vi "HFRR ADV v07.vi"() -> ()   [LabVIEW 2025] (continued)
, 1.5097292153342525, 1.5111107672344057, 1.5104967441676709, 1.5138738710347124, 1.5138738710347124, 1.5124923191345592, 1.5115712845344569, 1.510957261467722, 1.509422203800885, 1.5108037557010383, 1.5104967441676709, 1.5101897326343034, 1.5104967441676709, 1.5101897326343034, 1.5101897326343034, 1.5103432384009872, 1.5101897326343034, 1.5104967441676709, 1.5101897326343034, 1.5108037557010383, 1.5106502499343546, 1.5098827211009362, 1.5112642730010895, 1.5098827211009362, 1.510957261467722, 1.5104967441676709, 1.5101897326343034, 1.5101897326343034, 1.5103432384009872, 1.5108037557010383, 1.5097292153342525, 1.5111107672344057, 1.5108037557010383, 1.5104967441676709, 1.5112642730010895, 1.5103432384009872, 1.5097292153342525, 1.5104967441676709, 1.5106502499343546, 1.5108037557010383, 1.5100362268676197, 1.5106502499343546, 1.5106502499343546, 1.5103432384009872, 1.5097292153342525, 1.5106502499343546, 1.5100362268676197, 1.5111107672344057, 1.5108037557010383, 1.5100362268676197, 1.5101897326343034, 1.5117247903011406, 1.5117247903011406, 1.510957261467722, 1.5100362268676197, 1.510957261467722, 1.5112642730010895, 1.5103432384009872, 1.5112642730010895, 1.5098827211009362, 1.5112642730010895, 1.510957261467722, 1.5106502499343546, 1.5123388133678755, 1.5123388133678755, 1.5103432384009872, 1.5101897326343034, 1.5101897326343034, 1.5104967441676709, 1.5097292153342525, 1.5111107672344057, 1.5108037557010383, 1.5126458249012429, 1.5117247903011406, 1.5100362268676197, 1.5106502499343546, 1.5098827211009362, 1.5104967441676709, 1.5098827211009362, 1.5106502499343546, 1.5115712845344569, 1.5108037557010383, 1.5112642730010895, 1.5100362268676197, 1.5112642730010895, 1.5104967441676709, 1.5098827211009362, 1.5091151922675177, 1.5112642730010895, 1.5103432384009872, 1.514641399868131, 1.5154089287015495, 1.5117247903011406, 1.5111107672344057, 1.5101897326343034, 1.5098827211009362, 1.5106502499343546, 1.5106502499343546, 1.5106502499343546, 1.5106502499343546, 1.5104967441676709, 1.5112642730010895, 1.5103432384009872, 1.5108037557010383, 1.5106502499343546, 1.5097292153342525, 1.510957261467722, 1.5112642730010895, 1.5103432384009872, 1.510957261467722, 1.5112642730010895, 1.5111107672344057, 1.5106502499343546, 1.5097292153342525, 1.5101897326343034, 1.5097292153342525, 1.5114177787677732, 1.5100362268676197, 1.5103432384009872, 1.5114177787677732, 1.5104967441676709, 1.5112642730010895, 1.5108037557010383, 1.509422203800885, 1.5108037557010383, 1.510957261467722, 1.5108037557010383, 1.5108037557010383, 1.5106502499343546, 1.5108037557010383, 1.510957261467722, 1.5117247903011406, 1.5092686980342014, 1.5098827211009362, 1.5108037557010383, 1.5104967441676709, 1.510957261467722, 1.5111107672344057, 1.5114177787677732, 1.5114177787677732, 1.5114177787677732, 1.5100362268676197, 1.509422203800885, 1.5114177787677732, 1.5106502499343546, 1.5100362268676197, 1.5108037557010383, 1.5103432384009872, 1.5108037557010383, 1.510957261467722, 1.5101897326343034, 1.5103432384009872, 1.5098827211009362, 1.5114177787677732, 1.5108037557010383, 1.5104967441676709, 1.510957261467722, 1.5101897326343034, 1.5111107672344057, 1.5106502499343546, 1.5103432384009872, 1.5108037557010383, 1.5095757095675688, 1.5106502499343546, 1.5103432384009872, 1.5104967441676709, 1.5111107672344057, 1.5104967441676709, 1.5103432384009872, 1.5112642730010895, 1.5108037557010383, 1.5103432384009872, 1.5104967441676709, 1.5106502499343546, 1.5106502499343546, 1.5108037557010383, 1.5111107672344057, 1.5095757095675688, 1.5097292153342525, 1.5111107672344057, 1.5104967441676709, 1.5138738710347124, 1.5138738710347124, 1.5124923191345592, 1.5115712845344569, 1.510957261467722, 1.509422203800885, 1.5108037557010383, 1.5104967441676709, 1.5101897326343034, 1.5104967441676709, 1.5101897326343034, 1.5101897326343034, 1.5103432384009872, 1.5101897326343034, 1.5104967441676709, 1.5101897326343034, 1.5108037557010383, 1.5106502499343546, 1.5098827211009362, 1.5112642730010895, 1.5098827211009362, 1.510957261467722, 1.5104967441676709, 1.5101897326343034, 1.5101897326343034, 1.5103432384009872, 1.5108037557010383, 1.5097292153342525, 1.5111107672344057, 1.5108037557010383, 1.5104967441676709, 1.5112642730010895, 1.5103432384009872, 1.5097292153342525, 1.5104967441676709, 1.5106502499343546, 1.5108037557010383, 1.5100362268676197, 1.5106502499343546, 1.5106502499343546, 1.5103432384009872, 1.5097292153342525, 1.5106502499343546, 1.5100362268676197, 1.5111107672344057, 1.5108037557010383, 1.5100362268676197, 1.5101897326343034, 1.5117247903011406, 1.5117247903011406, 1.510957261467722, 1.5100362268676197, 1.510957261467722, 1.5112642730010895, 1.5103432384009872, 1.5112642730010895, 1.5098827211009362, 1.5112642730010895, 1.510957261467722, 1.5106502499343546, 1.5123388133678755, 1.5123388133678755, 1.5103432384009872, 1.5101897326343034, 1.5101897326343034, 1.5104967441676709, 1.5097292153342525, 1.5111107672344057, 1.5108037557010383, 1.5126458249012429, 1.5117247903011406, 1.5100362268676197, 1.5106502499343546, 1.5098827211009362, 1.5104967441676709, 1.5098827211009362, 1.5106502499343546, 1.5115712845344569, 1.5108037557010383, 1.5112642730010895, 1.5100362268676197, 1.5112642730010895, 1.5104967441676709, 1.5098827211009362, 1.5091151922675177, 1.5112642730010895, 1.5103432384009872, 1.514641399868131, 1.5154089287015495, 1.5117247903011406, 1.5111107672344057, 1.5101897326343034, 1.5098827211009362, 1.5106502499343546, 1.5106502499343546, 1.5106502499343546, 1.5106502499343546, 1.5104967441676709, 1.5112642730010895, 1.5103432384009872, 1.5108037557010383, 1.5106502499343546, 1.5097292153342525, 1.510957261467722, 1.5112642730010895, 1.5103432384009872, 1.510957261467722, 1.5112642730010895, 1.5111107672344057, 1.5106502499343546, 1.5097292153342525, 1.5101897326343034, 1.5097292153342525, 1.5114177787677732, 1.5100362268676197, 1.5103432384009872, 1.5114177787677732, 1.5104967441676709, 1.5112642730010895, 1.5108037557010383, 1.509422203800885, 1.5108037557010383, 1.510957261467722, 1.5108037557010383, 1.5108037557010383, 1.5106502499343546, 1.5108037557010383, 1.510957261467722, 1.5117247903011406, 1.5092686980342014, 1.5098827211009362, 1.5108037557010383, 1.5104967441676709, 1.510957261467722, 1.5111107672344057, 1.5114177787677732, 1.5114177787677732, 1.5114177787677732, 1.5100362268676197, 1.509422203800885, 1.5114177787677732, 1.5106502499343546, 1.5100362268676197, 1.5108037557010383, 1.5103432384009872, 1.5108037557010383, 1.510957261467722, 1.5101897326343034, 1.5103432384009872, 1.5098827211009362, 1.5114177787677732, 1.5108037557010383, 1.5104967441676709, 1.510957261467722, 1.5101897326343034, 1.5111107672344057, 1.5106502499343546, 1.5103432384009872, 1.5108037557010383, 1.5095757095675688, 1.5106502499343546, 1.5103432384009872, 1.5104967441676709, 1.5111107672344057, 1.5104967441676709, 1.5103432384009872, 1.5112642730010895, 1.5108037557010383, 1.5103432384009872, 1.5104967441676709, 1.5106502499343546, 1.5106502499343546, 1.5108037557010383, 1.5111107672344057, 1.5095757095675688, 1.5097292153342525, 1.5111107672344057, 1.5104967441676709, 1.5138738710347124, 1.5138738710347124, 1.5124923191345592, 1.5115712845344569, 1.510957261467722, 1.509422203800885, 1.5108037557010383, 1.5104967441676709, 1.5101897326343034, 1.5104967441676709, 1.5101897326343034, 1.5101897326343034, 1.5103432384009872, 1.5101897326343034, 1.5104967441676709, 1.5101897326343034, 1.5108037557010383, 1.5106502499343546, 1.5098827211009362, 1.5112642730010895, 1.5098827211009362, 1.510957261467722, 1.5104967441676709, 1.5101897326343034, 1.5101897326343034, 1.5103432384009872, 1.5108037557010383, 1.5097292153342525, 1.5111107672344057, 1.5108037557010383, 1.5104967441676709, 1.5112642730010895, 1.5103432384009872, 1.5097292153342525, 1.5104967441676709, 1.5106502499343546, 1.5108037557010383, 1.5100362268676197, 1.5106502499343546, 1.5106502499343546, 1.5103432384009872, 1.5097292153342525, 1.5106502499343546, 1.5100362268676197, 1.5111107672344057, 1.5108037557010383, 1.5100362268676197, 1.5101897326343034, 1.5117247903011406, 1.5117247903011406, 1.510957261467722, 1.5100362268676197, 1.510957261467722, 1.5112642730010895, 1.5103432384009872, 1.5112642730010895, 1.5098827211009362, 1.5112642730010895, 1.510957261467722, 1.5106502499343546, 1.5123388133678755, 1.5123388133678755, 1.5103432384009872, 1.5101897326343034, 1.5101897326343034, 1.5104967441676709, 1.5097292153342525, 1.5111107672344057, 1.5108037557010383, 1.5126458249012429, 1.5117247903011406, 1.5100362268676197, 1.5106502499343546, 1.5098827211009362, 1.5104967441676709, 1.5098827211009362, 1.5106502499343546, 1.5115712845344569, 1.5108037557010383, 1.5112642730010895, 1.5100362268676197, 1.5112642730010895, 1.5104967441676709, 1.5098827211009362, 1.5091151922675177, 1.5112642730010895, 1.5103432384009872, 1.514641399868131, 1.5154089287015495, 1.5117247903011406, 1.5111107672344057, 1.5101897326343034, 1.5098827211009362, 1.5106502499343546, 1.5106502499343546, 1.5106502499343546, 1.5106502499343546, 1.5104967441676709, 1.5112642730010895, 1.5103432384009872, 1.5108037557010383, 1.5106502499343546, 1.5097292153342525, 1.510957261467722, 1.5112642730010895, 1.5103432384009872, 1.510957261467722, 1.5112642730010895, 1.5111107672344057, 1.5106502499343546, 1.5097292153342525, 1.5101897326343034, 1.5097292153342525, 1.5114177787677732, 1.5100362268676197, 1.5103432384009872, 1.5114177787677732, 1.5104967441676709, 1.5112642730010895, 1.5108037557010383, 1.509422203800885, 1.5108037557010383, 1.510957261467722, 1.5108037557010383, 1.5108037557010383, 1.5106502499343546, 1.5108037557010383, 1.510957261467722, 1.5117247903011406, 1.5092686980342014, 1.5098827211009362, 1.5108037557010383, 1.5104967441676709, 1.510957261467722, 1.5111107672344057, 1.5114177787677732, 1.5114177787677732, 1.5114177787677732, 1.5100362268676197, 1.509422203800885, 1.5114177787677732, 1.5106502499343546, 1.5100362268676197, 1.5108037557010383, 1.5103432384009872, 1.5108037557010383, 1.510957261467722, 1.5101897326343034, 1.5103432384009872, 1.5098827211009362, 1.5114177787677732, 1.5108037557010383, 1.5104967441676709, 1.510957261467722, 1.5101897326343034, 1.5111107672344057, 1.5106502499343546, 1.5103432384009872, 1.5108037557010383, 1.5095757095675688, 1.5106502499343546, 1.5103432384009872, 1.5104967441676709, 1.5111107672344057, 1.5104967441676709, 1.5103432384009872, 1.5112642730010895, 1.5108037557010383, 1.5103432384009872, 1.5104967441676709, 1.5106502499343546, 1.5106502499343546, 1.5108037557010383, 1.5111107672344057, 1.5095757095675688, 1.5097292153342525, 1.5111107672344057, 1.5104967441676709, 1.5138738710347124, 1.5138738710347124, 1.5124923191345592, 1.5115712845344569, 1.510957261467722, 1.509422203800885, 1.5108037557010383, 1.5104967441676709, 1.5101897326343034, 1.5104967441676709, 1.5101897326343034, 1.5101897326343034, 1.5103432384009872, 1.5101897326343034, 1.5104967441676709, 1.5101897326343034, 1.5108037557010383, 1.5106502499343546, 1.5098827211009362, 1.5112642730010895, 1.5098827211009362, 1.510957261467722, 1.5104967441676709, 1.5101897326343034, 1.5101897326343034, 1.5103432384009872, 1.5108037557010383, 1.5097292153342525, 1.5111107672344057, 1.5108037557010383, 1.5104967441676709, 1.5112642730010895, 1.5103432384009872, 1.5097292153342525, 1.5104967441676709, 1.5106502499343546, 1.5108037557010383, 1.5100362268676197, 1.5106502499343546, 1.5106502499343546, 1.5103432384009872, 1.5097292153342525, 1.5106502499343546, 1.5100362268676197, 1.5111107672344057, 1.5108037557010383, 1.5100362268676197, 1.5101897326343034, 1.5117247903011406, 1.5117247903011406, 1.510957261467722, 1.5100362268676197, 1.510957261467722, 1.5112642730010895, 1.5103432384009872]
  out "Numeric":i32=178
  out "Flag":dbl format="%.2f"
  in  "Tab Control 3":enum32{"RMS", "LIVE"}(tab)
  out "array w/ subset deleted":dbl[](array[numeric])
  out "REMARKS":string="@WINDUCOM : RECIPROCATORY TEST RIG    DEFINITON FILE       \r  Sample ID :- , Load :-  2.00 N , Remarks :- , Date :- 05/11/2016, 06:04\r"
  out "Time 2":dbl=0.0004
  in  "reinit":bool=TRUE
  in  "Remarks : 2":string
  out "Err Count":i32
  out "PID-out":dbl
  out "Rate":dbl=2500.0 caption="Rate (Hz)" min=100.0 max=10000.0 step=1.0
  out "COUNT":i32
  out "FRICVALZ":dbl
  out "Sensor mean 3":dbl
  out "Sensor mean":dbl(slide) min=0.0 max=5.0 step=0.001 scale=0.0..5.0
  out "Sensor mean 2":dbl
  in  "ao0":errorcluster
  out "String 2":string
  out "clk":dbl min=0.0 max=999999999.0 step=0.25 format="%.2f"
  out "spm":string
  out "stp":dbl=0.25 min=0.25 max=60.0 step=0.25 format="%.2f"
  # "Start test and end test log--- done\nDisable heater ON and Humidity ON during the test --- done\ntemprature and ---done\nhumidity reach log\nauto start run true logic and log\nmanual start log once"
  # "System Control Commands\nS;1 - Starts the full automation cycle (Runs Priming-humidify till 70RH sequence first, then switches to Maintenance).\nS;0 - Stops the system immediately and enters Standby mode (Safe State: All actuators OFF).\nM;1 - Skips the priming sequence and jumps directly to Maintenance mode (PID control).\nR;1 - Resets the logic state machine and clears all errors, returning to Standby.\nService Mode (Manual Control)\nX;1 - Enters Manual Service Mode. This disables all automatic logic, sensor safety checks, and timers.\nX;0 - Exits Manual Service Mode and returns to Standby (Safe State).\nActuator Commands (Only work after sending X;1)\nP;[0-255] - Sets the Pump PWM. Note that this is Active Low (0 = Max Flow, 255 = Pump OFF).\nF;I;[0-255] - Sets the Intake Fan speed (0 = OFF, 255 = Max Speed).\nF;O;[0-255] - Sets the Exhaust Fan speed (0 = OFF, 255 = Max Speed).\nD;1 - Turns the Dehumidifier Relay ON.\nD;0 - Turns the Dehumidifier Relay OFF."
  # "°"
  # "HFRR adv"
  # "HFRR adv"
  # "Camera Initialization in Progress"
  # "Test Setup"
  # "SAMPLE INFO"
  # "Hz"
  # "N"
  # "mm"
  # "°C"
  # "%RH"
  # "min"
  # "mins remaining"
  # "%RH"
  # "°C"
  # "Coefficient of Friction"
  # "Frictional Force ( N )"
  # "Electrical Contact Resistance ( % )"
  # "Temperature ( °C )"
  # "Heater"
  # "( mm )"
  # "Hz"
  # "%Rh"
  # "Stroke ( mm )"
  # "Controller"
  # "%"
  # "N"
  # "deg C"
  # "N"
  # "Automated Scar Detection in Progress"
  # "Zoom Factor"
  # "%"
  # "Tools"
  # "Wear Scar Measurements"
  # "Wear Scar"
  # "Wear Scar"
  # "Wear Scar"
  # "µm"
  # "µm"
  # "µm"
  # "LAB-IQ\\ WO 2465 \\ v07 \\ April 2026"
  # "Data points"
  # "Captured if Stroke is +-0.5 of 1mm"
  # "Stroke calibration Procedure: \n1. Insert step 1 in between pushrod and stud and correct the offeset        value  of high pricision laser displacement sensor and the software value.\n2. Insert step 2 (of 0.5mm) and press the capture button to enter\nthe readings in the table shown below\n3. Follow the procedure 3 times and capture the values in  the table.\n4. Press Calculate button to read the error in the gain value."
  # "Calibration assembly image"
  # "ISO : WS1.4"
  # "Reference Fluid Information"
  # "Note:\nMake sure to place all images in the folder \"C:\\WinDucom\\im\" before clicking on \"Import Image.\""
  # "NOTE:\nPlace all the images in the path \"C:\\WinDucom\\im\" before clicking on Import Image"
  # "Wear Scar Measurements"
  # "Reference Fluid Information"
  # "Graph :"
types:
  T1 = typedef "Auto Start enum.ctl" = enum16{"Init", "Humidity & Temperature On", "Reach point", "Maintain Stage", "Start Stage", "close", "Exit"}
  T2 = enum32{"Home", "Dashboard", "Imaging", "Report", "Analysis", "About", "Test Setup"}
  T3 = enum32{"HOME", "Test Setup", "Acquire", "Adv Scar", "Adv Scar Report", "Compare Files", "About", "Advance", "Mooha"}
  T4 = enum16{"ASTM D6079", "ISO 12156", "CEC F-096-A-06", "Custom"}
  T5 = enum32{"Dashboard 1", "Dashboard 2", "Dashboard 3"}
  T6 = enum32{"COF", "Friction", "ECR", "Temperature", "Humidity", "Stroke"}
  T7 = enum32{"Coefficient Of Friction", "Air Temperature", "Humidity", "Stroke", "Sample Temperature", "Electrical Contact Resistance", "Frequency", "Air Temp vs Rh"}
  T8 = enum32{"Stroke Data", "Temperature Calibration", "Friction Force Raw Data"}
  T9 = cluster{"Proportional Gain (Kc)":dbl, "Integral Time (Ti, min)":dbl, "Derivative Time (Td, min)":dbl}
  T10 = enum32{"Freqz control", "Low Speed Analog Inputs & Digital IOs", "Temperature Tuning", "Voltage LVDT raw", "High Speed Analog Inputs - Displacement & Friction", "LVDT Calibration", "Sericve", "Friction Force Calibration", "Bytes At Port", "Loadcell Board"}
  T11 = cluster{"proportional gain (Kc)":dbl, "integral time (Ti, min)":dbl, "derivative time (Td, min)":dbl}
  T12 = typedef "imagedata.ctl" = cluster{"image type":i32, "image depth":i32, "image":u8[], "mask":u8[], "colors":u32[], "Rectangle":cluster{"left":i16, "top":i16, "right":i16, "bottom":i16}}
  T13 = enum32{"HOME", "Test Setup", "Acquire", "Compare Files", "Print Report", "About", "Advance", "Mooha"}
  T14 = cluster{"Read Heave and Surge":string, "Bytes at Heave Port":dbl, "Heave and Surge COM Port:":refnum<visa-resource-name>, "Com Port 2":refnum<visa-resource-name>, "Residual Due":string, "Heave COM Status 2":bool, "Heave COM Status":bool, "Port 2":bool, "Sway PPR":dbl, "Surge PPR":dbl, "Heave PPR":dbl, "Sway Pitch":dbl, "Surge Pitch":dbl, "Heave Pitch":dbl, "Sway Pulses/mm":dbl, "Surge Pulses/mm":dbl, "Heave Pulses/mm":dbl, "inner loop":dbl, "Read Heave and Surge 2":string, "String 36":string, "Write S":bool, "WriteCC1":string[], "Heave COM Loop":i32, "LastCom":string, "EXIT":bool, "Error Heave":errorcluster}
  T15 = enum8{"Enabled", "Disabled", "Disabled and Grayed Out"}
  T16 = typedef "POST ANALYSIS ENUM.ctl" = enum16{"OPEN EXE", "INIT", "OPEN FILE", "FIT", "DRAW REC", "DRAW LINE", "PAN", "ZOOM IN", "ZOOM OUT", "SET ZOOM", "CLEAR ROI", "GET MEASUREMENTS", "RESIZE MODE", "STREAM START", "STREAM STOP", "SHOW UI", "MINIMIZE UI", "HIDE UI", "CKISE APP", "CLOSE CONNECTION", "SAVE IMAGE", "SET ROI COLOR", "READ", "TCP CHECK", "CLOSE"}
  T17 = typedef "CAMERA LIVE FEED ENUM.ctl" = enum16{"OPEN EXE", "INIT", "READ", "CAMERA CONNECT", "CAMERA START", "CAMERA STOP", "CAMERA GRAY", "CAMERA RGB", "CAMERA MINIMIZE", "CAMERA CLOSE", "CAMERA MODE LIST", "CAMERA MODE SET", "CAMERA RESTORE", "CAMERA SAVE", "CLOSE"}
  T18 = cluster{"File Name":string, "Test Method":string, "Operator":string, "Fuel Description":string, "Date and time":string}
  T19 = enum32{"HOME", "Test Setup", "Acquire", "Compare Files", "About", "Advance", "Mooha"}
  T20 = enum16{"deny read/write", "deny write-only", "deny none"}
  T21 = typedef "NI_ReportGenerationCore.lvlib/HTML Report Image Alignment.ctl" = enum16{"(default)", "LEFT", "RIGHT", "TOP", "TEXTTOP", "MIDDLE", "ABSMIDDLE", "BASELINE", "BOTTOM", "ABSBOTTOM"}
  T22 = enum16{"open", "replace", "create", "open or create", "replace or create", "replace or create with confirmation"}
  T23 = enum16{"INIT", "READ", "MANUAL WRITE", "WRITE", "CLOSE", "ERROR INIT"}
  T24 = enum16{"open", "open or create", "create or replace", "create", "open (read only)"}
  T25 = cluster{"Mode":enum16{"RTU", "ASCII"}, "Slave Address":u8}
diagram:
  w2 = FALSE ("Visible")
  w6 = FALSE ("Humidity Off Command")
  w21 = "" ("USER ID")
  # "[CH1]    - FF\n[CH2]   - TEMPERATURE\n[CH3]    - Humidity\n[CH4]    - AIR TEMP\n[CH5]\\- Visa Uno\n[CH6] \\- Visa Due\n[CH7]  \\- file path\n[CH8]   - Displacement Gain\n[CHA]   - Stroke Gain\n[CHB]   - Stroke PID Gain\n[CHC]   -Language Selection\n[CHD]   -Power +\n[CHE]   -Power_\n[CHF]   -Heater\n[CHG]   -Humidity Wet\n[CHH]   -Humidity Dry\n[CHI]   -Integral Time \n[CHIJ   -Air intercept\n[CHI]   -Temp Intercept"
  n1 = flat-sequence {
    tunnel: [w59] -> w11
    tunnel: w11 -> [w73]
    tunnel: [w72] -> w10
    tunnel: ["ao0"] -> w13
    tunnel: w10 -> [_]
    tunnel: w13 -> [w138]
    tunnel: [w138] -> w12
    tunnel: w12 -> [w191]
    tunnel: [w189] -> w25
    tunnel: [w191] -> w24
    tunnel: w25 -> [w242]
    tunnel: w24 -> [w198]
    tunnel: [w242] -> w9
    tunnel: [w204] -> w8
    tunnel: [w192] -> w7
    tunnel: [w249] -> _
    tunnel: [w248] -> _
    tunnel: [w250] -> w53
    tunnel: w9 -> [w250]
    tunnel: w8 -> [w248]
    tunnel: w7 -> [w249]
    frame #0 {
      n2 = call "CLOSE CONNECTION.vi"("error in (no error)"="error in (no error) 2") -> ("error out"=w57:errorcluster)  [unwired: 10 in]
      n3 = call <vilib>:"Clear Errors.vi"("error in (no error)"=w57) -> ("error out"=w56:errorcluster)  [unwired: 5 in, 1 out]
      n4 = disable-structure shown="Enabled" {
        disable-tunnel: w56 -> [w63 _]
        disable-tunnel: [w62 _] -> w59
        frame Enabled {
          n5 = call <userlib>:"Fit VI window to Largest Dec.vi"("error in (no error)"=w63, "border spacing (2 px)"=1) -> ("error out"=w66:errorcluster, "dup VI Ref"=w70:refnum<vi>)  [unwired: 4 in]
          n6 = invoke on="Invoke Node" class="VI" method="FP.Run-Time Position.Maximized"(reference=w70, error in=w66) -> (error out=w67:errorcluster)  [unwired: 2 in, 3 out]
          n7 = call <vilib>:"Clear Errors.vi"("error in (no error)"=w67) -> ("error out"=w69:errorcluster)  [unwired: 5 in, 1 out]
          n8 = control-ref of="This VI"() -> (w61:refnum<vi>)
          n9 = invoke on="Invoke Node" class="VI" method="Default Vals.Reinit All"(reference=w61, error in=w69) -> (reference out=w65:refnum<vi>, error out=w64:errorcluster)  [unwired: 1 in, 1 out]
          n10 = Close Reference(reference=w65, error in (no error)=w64) -> (error out=w62:errorcluster)
        }
        frame Disabled {
        }
      }
      n11 = local write "sign in temp"(FALSE ("sign in temp")) -> ()
      n12 = property on="Sign In" class="Bool (strict)"("DisabledEnum"=T15."Disabled" ("Disabled")) -> ()  [unwired: 2 in, 2 out]
      n13 = property on="Auto Scar Check" class="Clust (strict)"("Visible"=TRUE) -> ()  [unwired: 2 in, 2 out]
    }
    frame #1 {
      n14 = call "dialog box.vi"("Status"="Before starting the test, verify that the microscope cable is connected.", "error in"=w73) -> ("error out"=w72:errorcluster)  [unwired: 8 in]
    }
    frame #2 {
      w80 = FALSE ("Upld AR 2")
      # "kkkkk"
      # "C:\\Windows\\wndcm_pw_stdED hfrr.txt"
      # "C:\\LAB-IQ NXT"
      # "C:\\LAB-IQ NXT\\wndcm_pw_stdED hfrr.txt"
      # "password file"
      n15 = Current VI's Path() -> (path=w93:path)
      n16 = Strip Path(path=w93) -> (stripped path=w86:path)  [unwired: 1 out]
      n17 = Path To String(path=w86) -> (string=w88:string)
      n18 = local write "conststatus"(0.0 ("rpm value : 2")) -> ()
      n19 = local write "Upld AR 2"(TRUE ("Upld AR 2")) -> ()
      n20 = local write "Lan flag"(0.0 ("Lan flag")) -> ()
      n21 = local write "COUNT"(0 ("COUNT")) -> ()
      n22 = local write "FLAG 2"(0.0 ("FLAG 2")) -> ()
      n23 = local write "Com flag"(u32 0 ("Com flag")) -> ()
      n24 = local write "Re-Initialise"(TRUE ("Re-Initialise")) -> ()
      n25 = local write "refresh flag"(FALSE ("refresh flag")) -> ()
      n26 = local write "Json St Flg"(w80) -> ()
      n27 = Search/Split String(string=w88, search string/char (-)=".exe") -> (match + rest of string=w90:string)  [unwired: 1 in, 2 out]
      n28 = Match True/False String(2:".vi" ("false string"), 3:".exe" ("true string"), 4:w90) -> (0:w87:bool)  [unwired: 1 out]
      n29 = local write "Json End Flg"(w80) -> ()
      n30 = case shown="True" w87 {
        tunnel: w86 -> [w109 w111]
        tunnel: [w109 w110] -> w84
        frame False {
        }
        frame True {
          n31 = Strip Path(path=w111) -> (stripped path=w110:path)  [unwired: 1 out]
        }
      }
      n32 = Path To String(path=w84) -> (string=→"Gain path":string)
      n33 = local write "Main Tab Display"(T5."Dashboard 1" ("Main Tab Display")) -> ()
      n34 = local write "main tab sub"(enum32{"Page 1", "Page 2"}."Page 1" ("main tab sub")) -> ()
      n35 = local write "Main Tab"(T3."HOME" ("Main Tab")) -> ()
      n36 = local write "EVENT LOG"("") -> ()
      n37 = List Folder(path=path "C:/LAB-IQ" ("directory path"), pattern="*.txt") -> (filenames=w99:string[])  [unwired: 2 in, 3 out]
      n38 = Search 1D Array(1D array=w99, element="wndcm_pw_stdED hfrr.txt") -> (index of element=w102:i32)  [unwired: 1 in]
      n39 = Equal?(x=w102, y=-1) -> (x = y?=w97:bool)
      n40 = case shown="True" w97 {
        frame False {
        }
        frame True {
          n41 = String To Byte Array(string="123\n") -> (unsigned byte array=w116:u8[])
          n42 = Array Size(array=w116) -> (size(s)=w115:i32)
          n43 = for {
            N: w115 -> [_]
            tunnel: w116 -> [w129]
            tunnel: [w126] -> w118 mode=indexing
            tunnel: w115 -> [w121]
            i -> [w119]
            n44 = Decrement(x=w121) -> (x-1=w122:i32)
            n45 = Equal?(x=w119, y=w122) -> (x = y?=w123:bool)
            n46 = Index Array(array=w129, index=w119) -> (element=w128:u8)
            n47 = Number To Decimal String(number=w128) -> (decimal integer string=w127:string)  [unwired: 1 in]
            n48 = Select(t="", s=w123, f="\r") -> (s? t:f=w120:string)
            n49 = Concatenate Strings(w127, w120) -> (w126:string)
          }
          n50 = local read "file path"() -> (w112:path)
          n51 = Concatenate Strings(w118) -> (w114:string)
          n52 = call <vilib>:"Write Characters To File.vi"("append to file? (new file:F)"=FALSE, "character string"=w114, "file path (dialog if empty)"=w112) -> ()  [unwired: 2 in, 1 out]
        }
      }
      n53 = local write "clk"(0.0 ("clk")) -> ()
      n54 = local write "Flag"(0.0 ("Flag")) -> ()
      "file path" <- path "C:/LAB-IQ/wndcm_pw_stdED hfrr.txt" ("file path")
      "FF buffer" <- dbl[] [] ("FF buffer")
    }
    frame #3 {
      # "C:\\WinDucom\\calibrate WO 2391.dcf"
      n55 = String To Path(string="C:\\LAB-IQ\\calibrate WO 2465.dcf") -> (path=w137:path)
      n56 = Open/Create/Replace File "Open File"(file path (use dialog)=w137) -> (refnum out=w136:refnum<file>)  [unwired: 5 in, 2 out]
      n57 = for {
        N: 24 -> [_]
        tunnel: w136 -> [w157]
        i -> [w151]
        (unwired) TRUE ("line mode (F)")
        n58 = Read from Text File "Read File"(file (use dialog)=w157) -> (text=w156:string)  [unwired: 3 in, 3 out]
        n59 = Match Pattern(string=w156, regular expression="]") -> (after substring=w154:string)  [unwired: 1 in, 3 out]
        n60 = String Subset(string=w156, offset (0)=5, length (rest)=10 ("length (rest)")) -> (substring=w149:string)
        n61 = Fract/Exp String To Number(string=w149) -> (number=w150:dbl)  [unwired: 3 in, 1 out]
        n62 = Match Pattern(string=w154, regular expression="-") -> (before substring=w152:string)  [unwired: 1 in, 3 out]
        n63 = case shown="7" w151 {
          tunnel: w150 -> [w160 w161 w162 w163 _ _ _ w168 w169 w170 w173 w174 w175 w176 w177 w178 w179 w182 w183 _ _ w186 _ _ _]
          tunnel: w152 -> [_ _ _ _ w164 w165 w166 _ _ _ _ _ _ _ _ _ _ _ _ w184 w185 _ w187 w188 _]
          frame 0 {
            n64 = local write "FRIC. FORCE :"(w160) -> ()
          }
          frame 1 {
            n65 = local write "TEMPERATURE :"(w161) -> ()
          }
          frame 2 {
            n66 = local write "HUMIDITY:"(w162) -> ()
          }
          frame 3 {
            n67 = local write "AIR TEMPERATURE :"(w163) -> ()
          }
          frame 4 {
            n68 = local write "Com Port 1"(w164) -> ()
          }
          frame 5 {
            n69 = local write "Com Port 2"(w165) -> ()
            n70 = local write "visa due"(w165) -> ()
          }
          frame 6 {
            n71 = String To Path(string=w166) -> (path=w167:path)
            n72 = local write "File Path"(w167) -> ()
          }
          frame 7 {
            n73 = local write "DISPLACEMENT :"(w168) -> ()
          }
          frame 8 {
            n74 = local write "STROKE GAIN :"(w169) -> ()
          }
          frame 9 {
            n75 = local read "Stroke PID Gains"() -> (w172:T9)
            n76 = Bundle By Name(cluster=w172, "Proportional Gain (Kc)"=w170) -> (w171:T9)
            n77 = local write "Stroke PID Gains"(w171) -> ()
          }
          frame 10 {
            n78 = local write "Language Selection"(w173) -> ()
          }
          frame 11 {
            n79 = local write "CH-POWER +"(w174) -> ()
          }
          frame 12 {
            n80 = local write "CH-POWER -"(w175) -> ()
          }
          frame 13 {
            n81 = local write "CH-HEATER"(w176) -> ()
          }
          frame 14 {
            n82 = local write "CH-HUMIDITY WET"(w177) -> ()
          }
          frame 15 {
            n83 = local write "CH-HUMIDITY DRY"(w178) -> ()
          }
          frame 16 {
            n84 = local read "Stroke PID Gains"() -> (w181:T9)
            n85 = Bundle By Name(cluster=w181, "Integral Time (Ti, min)"=w179) -> (w180:T9)
            n86 = local write "Stroke PID Gains"(w180) -> ()
          }
          frame 17 {
            n87 = local write "AIR TEMP INTERCEPT:"(w182) -> ()
          }
          frame 18 {
            n88 = local write "TEMP INTERCEPT:"(w183) -> ()
          }
          frame 19 {
            n89 = local write "S.NO"(w184) -> ()
          }
          frame 20 {
            n90 = local write "Com Port 3"(w185) -> ()
          }
          frame 21 {
            n91 = local write "LvdtOff"(w186) -> ()
          }
          frame 22 {
            n92 = local write "Humidity :"(w187) -> ()
          }
          frame 23 {
            n93 = local write "Camera Port :"(w188) -> ()
          }
          frame 24, Default {
          }
        }
      }
      n94 = String To Path(string="C:\\LAB-IQ\\Image Calibrate v01.dcf") -> (path=w133:path)
      n95 = Open/Create/Replace File ("Open File")(file path (use dialog)=w133) -> (refnum out=w132:refnum<file>)  [unwired: 5 in, 2 out]
      n96 = for {
        N: 4 -> [_]
        tunnel: w132 -> [w144]
        i -> [w140]
        n97 = Read from Text File ("Read File")(file (use dialog)=w144) -> (text=w145:string)  [unwired: 3 in, 3 out]
        n98 = String Subset(string=w145, offset (0)=6, length (rest)=10 ("length (rest)")) -> (substring=w141:string)
        n99 = Fract/Exp String To Number(string=w141) -> (number=w139:dbl)  [unwired: 3 in, 1 out]
        n100 = case shown="3" w140 {
          tunnel: w139 -> [w146 w147 _ w148 _]
          frame 0 {
            n101 = local write "5x Gain"(w146) -> ()
          }
          frame 1 {
            n102 = local write "10x Gain"(w147) -> ()
          }
          frame 2 {
          }
          frame 3 {
            n103 = local write "100x gain"(w148) -> ()
          }
          frame 4, Default {
          }
        }
      }
    }
    frame #4 {
      n104 = Wait (ms)(milliseconds to wait=u32 1000) -> (millisecond timer value=w189:u32)
    }
    frame #5 {
      w207 = u32 2000 ("milliseconds to wait")
      w234 = u32 2000 ("milliseconds to wait")
      n105 = local read "Re-Initialise"() -> (w241:bool)
      n106 = case shown="True" w241 {
        frame False {
        }
        frame True {
          n107 = local write "Re-Initialise"(FALSE ("Re-Initialise")) -> ()
        }
      }
      n108 = call "CAMERA LIVE FEED FGV.vi"("Enum - Menu"=CAMERA_LIVE_FEED_ENUM."OPEN EXE", "error in (no error)"=w198) -> ("error out"=w240:errorcluster)  [unwired: 8 in, 1 out]
      n109 = call "Stall Data Flow.vim"("value in"=w240, "milliseconds to wait"=w234) -> ("value out"=w238:errorcluster)  [unwired: 1 out]
      n110 = call "CAMERA LIVE FEED FGV.vi"("Enum - Menu"=CAMERA_LIVE_FEED_ENUM."INIT", "error in (no error)"=w238) -> ("error out"=w236:errorcluster)  [unwired: 8 in, 1 out]
      n111 = call "IMAGE ANALYSIS.vi"("Enum"=POST_ANALYSIS_ENUM."OPEN EXE", "error in"=w198) -> ("error out"=w195:errorcluster)  [unwired: 8 in, 1 out]
      n112 = case shown="Error .." w236 {
        selector: w236 -> [w243 _]
        tunnel: [w243 _] -> w235
        frame No Error {
        }
        frame Error {
          n113 = One Button Dialog(message="Camera initialization error.\nPlease Restart the software") -> ()  [unwired: 1 in, 1 out]
        }
      }
      n114 = call "Stall Data Flow.vim"("value in"=w195, "milliseconds to wait"=u32 8000) -> ("value out"=w194:errorcluster)  [unwired: 1 out]
      n115 = property on="Camera Port :" class="CmbBox"() -> ("Strings[]"=w232:string[], "Value"=w233:string)  [unwired: 2 in, 2 out]
      n116 = call "IMAGE ANALYSIS.vi"("Enum"=POST_ANALYSIS_ENUM."INIT", "error in"=w194) -> ("error out"=w192:errorcluster)  [unwired: 8 in, 1 out]
      n117 = Search 1D Array(1D array=w232, element=w233) -> (index of element=w231:i32)  [unwired: 1 in]
      n118 = Type Cast(type=30, x=w231) -> (*(type *) &x=w229:i32)
      n119 = call "Stall Data Flow.vim"("value in"=w235, "milliseconds to wait"=w234) -> ("value out"=w211:errorcluster)  [unwired: 1 out]
      n120 = Add(x=w229, y=48) -> (x+y=w210:i32)
      n121 = call "CAMERA LIVE FEED FGV.vi"("Enum - Menu"=CAMERA_LIVE_FEED_ENUM."CAMERA CONNECT", "error in (no error)"=w211, "CAMERA PORT"=w210) -> ("error out"=w220:errorcluster)  [unwired: 7 in, 1 out]
      n122 = call "Stall Data Flow.vim"("value in"=w220, "milliseconds to wait"=u32 5000) -> ("value out"=w221:errorcluster)  [unwired: 1 out]
      n123 = call "CAMERA LIVE FEED FGV.vi"("Enum - Menu"=CAMERA_LIVE_FEED_ENUM."CAMERA MODE LIST", "error in (no error)"=w221) -> ("error out"=w223:errorcluster)  [unwired: 8 in, 1 out]
      n124 = call "Stall Data Flow.vim"("value in"=w223, "milliseconds to wait"=w207) -> ("value out"=w222:errorcluster)  [unwired: 1 out]
      n125 = Type Cast(type=30, x=0) -> (*(type *) &x=w203:i32)
      n126 = Add(x=w203, y=48) -> (x+y=w201:i32)
      n127 = call "CAMERA LIVE FEED FGV.vi"("Enum - Menu"=CAMERA_LIVE_FEED_ENUM."READ", "error in (no error)"=w222) -> ("error out"=w209:errorcluster, "data out"=→"data out":string)  [unwired: 8 in]
      n128 = call "Stall Data Flow.vim"("value in"=w209, "milliseconds to wait"=w207) -> ("value out"=w208:errorcluster)  [unwired: 1 out]
      n129 = call "CAMERA LIVE FEED FGV.vi"("Enum - Menu"=CAMERA_LIVE_FEED_ENUM."CAMERA MODE SET", "error in (no error)"=w208, "CAMERA MODE"=w201) -> ("error out"=w205:errorcluster)  [unwired: 7 in, 1 out]
      n130 = call "Stall Data Flow.vim"("value in"=w205, "milliseconds to wait"=u32 2000) -> ("value out"=w225:errorcluster)  [unwired: 1 out]
      n131 = call "CAMERA LIVE FEED FGV.vi"("Enum - Menu"=CAMERA_LIVE_FEED_ENUM."CAMERA START", "error in (no error)"=w225) -> ("error out"=w226:errorcluster)  [unwired: 8 in, 1 out]
      n132 = call "Stall Data Flow.vim"("value in"=w226, "milliseconds to wait"=u32 1000) -> ("value out"=w227:errorcluster)  [unwired: 1 out]
      n133 = call "CAMERA LIVE FEED FGV.vi"("Enum - Menu"=CAMERA_LIVE_FEED_ENUM."CAMERA MINIMIZE", "error in (no error)"=w227) -> ("error out"=w204:errorcluster)  [unwired: 8 in, 1 out]
    }
    frame #6 {
      n134 = case shown="No Error" w248 {
        frame No Error {
          n135 = property on="Auto Scar Check" class="Clust (strict)"("Visible"=FALSE) -> ()  [unwired: 2 in, 2 out]
        }
        frame Error {
        }
      }
      n136 = local write "sign in temp"(TRUE ("sign in temp")) -> ()
      n137 = property on="Sign In" class="Bool (strict)"("DisabledEnum"=T15."Enabled" ("Disabled")) -> ()  [unwired: 2 in, 2 out]
    }
  }
  n138 = property on="Auto Start Test" class="Bool (strict)"("Visible"=TRUE) -> ()  [unwired: 2 in, 2 out]
  n139 = while {
    shift-right: [w253] -> _
    shift-left: "Enum - Selector" -> [w254]
    stop <- w255 stop-if-true
    # "Auto Start Logic Loop"
    n140 = case shown="\"Reach point\"" w254 {
      tunnel: [w258 w264 w275 w307 w338 Auto_Start_enum."Exit" ("Enum - Selector") Auto_Start_enum."Init" ("Enum - Selector")] -> w253
      frame "Init", Default {
        n141 = local read "Auto Start Test"() -> (w257:bool)
        n142 = Select(t=Auto_Start_enum."Humidity & Temperature On" ("Enum - Selector"), s=w257, f=Auto_Start_enum."Init") -> (s? t:f=w258:T1)
      }
      frame "Humidity & Temperature On" {
        n143 = flat-sequence {
          tunnel: [Auto_Start_enum."Reach point" ("Enum - Selector")] -> w261
          frame #0 {
            w265 = T15."Disabled and Grayed Out" ("Disabled")
            w266 = TRUE ("Heater Button")
            n144 = property on="Humidity" class="Bool (strict)"("DisabledEnum"=w265) -> ()  [unwired: 2 in, 2 out]
            n145 = property on="Heater Button" class="Bool (strict)"("DisabledEnum"=w265) -> ()  [unwired: 2 in, 2 out]
            n146 = local write "Heater Button"(w266) -> ()
            n147 = local write "Humidity"(w266) -> ()
          }
          frame #1 {
            n148 = Wait (ms)(milliseconds to wait=u32 1000) -> ()  [unwired: 1 out]
          }
          frame #2 {
            n149 = local write "Reach point temp"(TRUE ("Reach point temp")) -> ()
          }
        }
        n150 = local read "Auto Start Test"() -> (w263:bool)
        n151 = Not(x=w263) -> (.not. x?=w262:bool)
        n152 = Select(t=Auto_Start_enum."close", s=w262, f=w261) -> (s? t:f=w264:T1)
      }
      frame "Reach point" {
        w276 = TRUE ("PAUSE")
        w284 = 1.0 ("y")
        w287 = 1.0 ("y")
        n153 = local read "Set Temperature:"() -> (w288:dbl)
        n154 = local read "Set Humidity:"() -> (w283:dbl)
        n155 = local read "Humidity ( %RH )"() -> (w289:dbl)
        n156 = Add(x=w288, y=w287) -> (x+y=w286:dbl)
        n157 = Subtract(x=w288, y=w287) -> (x-y=w285:dbl)
        n158 = Add(x=w283, y=w284) -> (x+y=w282:dbl)
        n159 = Subtract(x=w283, y=w284) -> (x-y=w281:dbl)
        n160 = local read "TEMP"() -> (w290:dbl)
        n161 = In Range and Coerce(upper limit=w282, x=w289, lower limit=w281) -> (In Range?=w270:bool)  [unwired: 1 out]
        n162 = In Range and Coerce(upper limit=w286, x=w290, lower limit=w285) -> (In Range?=w271:bool)  [unwired: 1 out]
        n163 = case shown="True" w270 {
          frame False {
          }
          frame True {
            n164 = case shown="True" "Reach point Humidity" {
              selector: "Reach point Humidity" -> [_ w296]
              frame False {
              }
              frame True {
                n165 = local read "EVENT LOG"() -> (w293:string)
                n166 = Not(x=w296) -> (.not. x?=w295:bool)
                n167 = local write "Reach point Humidity"(w295) -> ()
                n168 = call "Event Log.vi"("Content"="Target Humidity reached", "EVENT LOG"=w293) -> ("EVENT LOG"=w294:string)  [unwired: 8 in, 1 out]
                n169 = local write "EVENT LOG"(w294) -> ()
              }
            }
          }
        }
        n170 = case shown="True" w271 {
          frame False {
          }
          frame True {
            n171 = case shown="True" "Reach point temp" {
              selector: "Reach point temp" -> [_ w302]
              frame False {
              }
              frame True {
                n172 = local read "EVENT LOG"() -> (w299:string)
                n173 = Not(x=w302) -> (.not. x?=w301:bool)
                n174 = local write "Reach point temp"(w301) -> ()
                n175 = call "Event Log.vi"("Content"="Target Temperature reached", "EVENT LOG"=w299) -> ("EVENT LOG"=w300:string)  [unwired: 8 in, 1 out]
                n176 = local write "EVENT LOG"(w300) -> ()
              }
            }
          }
        }
        n177 = local read "Auto Start Test"() -> (w274:bool)
        n178 = And(x=w271, y=w270) -> (x .and. y?=w280:bool)
        n179 = Select(t=Auto_Start_enum."Maintain Stage" ("Enum - Selector"), s=w280, f=Auto_Start_enum."Reach point" ("Enum - Selector")) -> (s? t:f=w277:T1)
        n180 = Not(x=w274) -> (.not. x?=w273:bool)
        n181 = Select(t=Auto_Start_enum."close", s=w273, f=w277) -> (s? t:f=w275:T1)
        n182 = call "ELAPSED TIMER VI.vi"("RESET"=w276, "PAUSE"=w276) -> ()  [unwired: 7 in, 3 out]
      }
      frame "Maintain Stage" {
        w316 = 1.0 ("y")
        w315 = 1.0 ("y")
        # "Humidity and  temperatures Set Point  have been reached"
        n183 = local read "Set Temperature:"() -> (w322:dbl)
        n184 = local read "Set Humidity:"() -> (w319:dbl)
        n185 = local read "Humidity ( %RH )"() -> (w323:dbl)
        n186 = Add(x=w322, y=w315) -> (x+y=w321:dbl)
        n187 = Subtract(x=w322, y=w315) -> (x-y=w320:dbl)
        n188 = local read "TEMP"() -> (w324:dbl)
        n189 = Add(x=w319, y=w316) -> (x+y=w318:dbl)
        n190 = Subtract(x=w319, y=w316) -> (x-y=w317:dbl)
        n191 = In Range and Coerce(upper limit=w321, x=w324, lower limit=w320) -> (In Range?=w314:bool)  [unwired: 1 out]
        n192 = In Range and Coerce(upper limit=w318, x=w323, lower limit=w317) -> (In Range?=w313:bool)  [unwired: 1 out]
        n193 = And(x=w314, y=w313) -> (x .and. y?=w312:bool)
        n194 = Not(x=w312) -> (.not. x?=w311:bool)
        n195 = call "ELAPSED TIMER VI.vi"("TARGET"=60.0, "RESET"=w311, "PAUSE"=FALSE) -> ("ELAPSED INDICATION"=w308:bool)  [unwired: 6 in, 2 out]
        n196 = case shown="True" w308 {
          tunnel: w308 -> [_ w327]
          tunnel: [Auto_Start_enum."Maintain Stage" ("Enum - Selector") w326] -> w306
          frame False {
          }
          frame True {
            n197 = stacked-sequence {
              tunnel: w327 -> [_ _ _ _ _]
              tunnel: [_ _ _ _ Auto_Start_enum."Start Stage" ("Enum - Selector")] -> w326
              frame #0 {
                n198 = local read "EVENT LOG"() -> (w329:string)
                n199 = call "Event Log.vi"("Content"="Humidity and temperature set point has stabilized.", "EVENT LOG"=w329) -> ("EVENT LOG"=w330:string)  [unwired: 8 in, 1 out]
                n200 = local write "EVENT LOG"(w330) -> ()
              }
              frame #1 {
                n201 = Wait (ms)(milliseconds to wait=u32 100) -> ()  [unwired: 1 out]
              }
              frame #2 {
                n202 = local read "EVENT LOG"() -> (w333:string)
                n203 = call "Event Log.vi"("Content"="Auto Test Started", "EVENT LOG"=w333) -> ("EVENT LOG"=w334:string)  [unwired: 8 in, 1 out]
                n204 = local write "EVENT LOG"(w334) -> ()
              }
              frame #3 {
                w335 = TRUE ("RUN")
                n205 = local write "RUN"(w335) -> ()
                "Auto Start Temp" <- w335
              }
              frame #4 {
              }
            }
          }
        }
        n206 = local read "Auto Start Test"() -> (w305:bool)
        n207 = Not(x=w305) -> (.not. x?=w304:bool)
        n208 = Select(t=Auto_Start_enum."close", s=w304, f=w306) -> (s? t:f=w307:T1)
      }
      frame "Start Stage" {
        w337 = TRUE ("PAUSE")
        n209 = local read "Auto Start Test"() -> (w342:bool)
        n210 = Not(x=w342) -> (.not. x?=w341:bool)
        n211 = Select(t=Auto_Start_enum."close" ("Enum - Selector"), s=w341, f=Auto_Start_enum."Start Stage" ("Enum - Selector")) -> (s? t:f=w338:T1)
        n212 = call "ELAPSED TIMER VI.vi"("RESET"=w337, "PAUSE"=w337) -> ()  [unwired: 7 in, 3 out]
      }
      frame "close" {
        w343 = FALSE ("Heater Button")
        n213 = local write "RUN"(w343) -> ()
        n214 = local write "Heater Button"(w343) -> ()
        n215 = local write "Humidity"(w343) -> ()
        n216 = local write "Auto Start Test"(w343) -> ()
      }
      frame "Exit" {
      }
    }
    n217 = Wait (ms)(milliseconds to wait=u32 100) -> ()  [unwired: 1 out]
    n218 = local read "Quit"() -> (w255:bool)
  }
  n219 = while {
    stop <- w371 stop-if-true
    w354 = errorcluster {"status"=FALSE, "code"=0, "source"=""} ("error in (no error) 3")
    # "this loop is for manual report generation"
    n220 = local read "Confirm Measrurement"() -> (w353:bool)
    n221 = case shown="True" w353 {
      selector: w353 -> [_ w460]
      tunnel: errorcluster {"status"=FALSE, "code"=0, "source"=""} ("error in (no error) 3") -> [_ w461]
      tunnel: [_ w459] -> _
      frame False {
      }
      frame True {
        n222 = stacked-sequence {
          tunnel: w461 -> [_ w492 _]
          tunnel: w460 -> [_ _ w591]
          tunnel: [_ w480 _] -> w459
          frame #0 {
            n223 = String To Path(string="C:\\LAB-IQ\\Image Calibrate v01.dcf") -> (path=w464:path)
            n224 = Open/Create/Replace File ("Open File")(file path (use dialog)=w464) -> (refnum out=w465:refnum<file>)  [unwired: 5 in, 2 out]
            n225 = for {
              N: 4 -> [_]
              tunnel: w465 -> [w471]
              i -> [w467]
              n226 = Read from Text File ("Read File")(file (use dialog)=w471) -> (text=w472:string)  [unwired: 3 in, 3 out]
              n227 = String Subset(string=w472, offset (0)=6, length (rest)=10 ("length (rest)")) -> (substring=w468:string)
              n228 = Fract/Exp String To Number(string=w468) -> (number=w466:dbl)  [unwired: 3 in, 1 out]
              n229 = case shown="3" w467 {
                tunnel: w466 -> [w473 w474 _ w475 _]
                frame 0 {
                  n230 = local write "5x Gain"(w473) -> ()
                }
                frame 1 {
                  n231 = local write "10x Gain"(w474) -> ()
                }
                frame 2 {
                }
                frame 3 {
                  n232 = local write "100x gain"(w475) -> ()
                }
                frame 4, Default {
                }
              }
            }
          }
          frame #1 {
            n233 = local read "Magnification :"() -> (w485:string)
            n234 = case shown="\"10x\"" w485 {
              tunnel: [w527 w528] -> w483
              frame "5x", Default {
                n235 = local read "5x Gain"() -> (w527:dbl)
              }
              frame "10x" {
                # "5x"
                n236 = local read "10x Gain"() -> (w528:dbl)
              }
            }
            n237 = call "IMAGE ANALYSIS.vi"("Enum"=POST_ANALYSIS_ENUM."GET MEASUREMENTS", "error in"=w492) -> ("error out"=w499:errorcluster)  [unwired: 8 in, 1 out]
            n238 = call "Stall Data Flow.vim"("value in"=w499, "milliseconds to wait"=u32 1000) -> ("value out"=w498:errorcluster)  [unwired: 1 out]
            n239 = local read "Test File List :"() -> (w496:string)
            n240 = call "IMAGE ANALYSIS.vi"("Enum"=POST_ANALYSIS_ENUM."READ", "error in"=w498) -> ("error out"=w495:errorcluster, "data out"=w486:string)  [unwired: 8 in]
            n241 = Match Pattern(string=w486, regular expression="\"type\": ") -> (after substring=w490:string)  [unwired: 1 in, 3 out]
            n242 = call "IMAGE PATH CREATION PY.vi"("error in (no error)"=w495, "File Name :"=w496) -> ("error out"=w494:errorcluster, "File Path"=w482:path, "File Path String:"=w477:string)  [unwired: 7 in]
            n243 = Match Pattern(string=w490, regular expression=",") -> (before substring=w476:string)  [unwired: 1 in, 3 out]
            n244 = local read "Calibration Tab"() -> (w479:enum32{"Measrument", "Calibrate"})
            n245 = call "Stall Data Flow.vim"("value in"=w494, "milliseconds to wait"=u32 250) -> ("value out"=w478:errorcluster)  [unwired: 1 out]
            n246 = Equal?(x=w476, y="\"rectangle\"") -> (x = y?=w487:bool)
            n247 = case shown="False" w487 {
              tunnel: w486 -> [w533 w588]
              tunnel: w483 -> [_ w579]
              tunnel: cluster{"major":dbl, "minor":dbl, "average":dbl} {"major"=0.0, "minor"=0.0, "average"=0.0} -> [w531 w575]
              tunnel: [w530 w572] -> w481
              tunnel: w476 -> [w532 _]
              tunnel: w483 -> [w529 _]
              frame False {
                n248 = Equal?(x=w532, y="\"line\"") -> (x = y?=w534:bool)
                n249 = case shown="True" w534 {
                  tunnel: w533 -> [_ w549]
                  tunnel: w531 -> [w536 w548]
                  tunnel: [w536 w546] -> w530
                  tunnel: w529 -> [_ w545]
                  frame False {
                  }
